vi "wariancja i odchylenie.vi"(10 "Array":dbl[](array[numeric]), 11 "Liczba probek":i32) -> (2 "Odchylenie\nstandardowe":dbl, 3 "Wariancja":dbl)   [LabVIEW 2019]
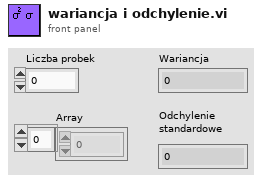
[diagram p1: front panel]
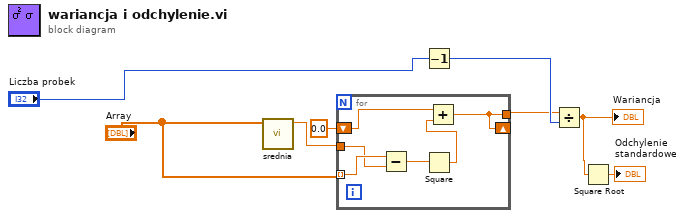
[diagram p0: block diagram]
diagram:
  n1 = call "srednia.vi"("Array"="Array") -> ("Srednia"=w1:dbl)  [unwired: 8 in, 2 out]
  n2 = for {
    tunnel: "Array" -> [w14] mode=indexing
    tunnel: w1 -> [w13]
    shift-right: [w9] -> _
    shift-left: 0.0 -> [w11]
    tunnel: [w9] -> w2
    n3 = Subtract(x=w14, y=w13) -> (x-y=w12:dbl)
    n4 = Square(x=w12) -> (x^2=w10:dbl)
    n5 = Add(x=w11, y=w10) -> (x+y=w9:dbl)
  }
  n6 = Decrement(x="Liczba probek") -> (x-1=w7:i32)
  n7 = Divide(x=w2, y=w7) -> (x/y=w3:dbl)
  "Wariancja" <- w3
  n8 = Square Root(x=w3) -> (sqrt(x)=→"Odchylenie\nstandardowe":dbl)
